vi "Microscopy.Acquisition Engine.vi"(5 "Acquisition Parameters":T4, 6 "Trig Offset":u8, 7 "Reset?":bool, 8 "Data Valid In":bool, 9 "Reference Trigger Edge?":bool, 10 "Arm Acquisition Engine":bool, 11 "Channel Data In":T3=[0, 0, 0, 0]) -> (0 "Data Valid Out":bool, 1 "Read from Buffer":bool, 2 "Acquisition Status":T1={"Reset"=FALSE, "Acquisition Engine Start (Arm)"=FALSE, "Current State"=enum."Acquire Pre-Trigger Samples", "Trig Offset"=0, "Points Unread"=0, "Points Acquired"=0, "Records Done"=0, "Start of Read"=FALSE, "End of Read"=FALSE, "Start of Record"=FALSE, "End of Record"=FALSE, "Ready for Ref Trig"=FALSE, "In Reset?"=FALSE}, 3 "Channel Data Out":T3, 4 "Ready for Ref Trig":bool)   [LabVIEW 2012]
doc: "This VI executes the state machine of the acquisition engine."
uses:
  Acquisition Parameters.ctl
  Multi-Channel Analog Input Data.ctl
  Acquisition Status.ctl
  Acquisition Engine State.ctl
panel:
  in  "Re-Arm Ticks to Wait":u16=3
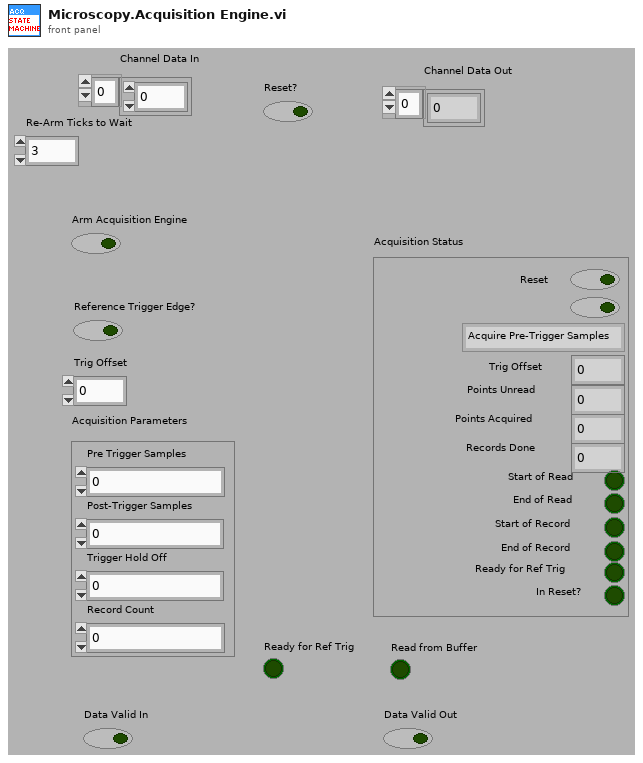
[diagram p1: front panel]
types:
  T1 = typedef "Acquisition Status.ctl" = cluster{"Reset":bool, "Acquisition Engine Start (Arm)":bool, "Current State":T2, "Trig Offset":u8, "Points Unread":u16, "Points Acquired":u16, "Records Done":u16, "Start of Read":bool, "End of Read":bool, "Start of Record":bool, "End of Record":bool, "Ready for Ref Trig":bool, "In Reset?":bool}
  T2 = typedef "Acquisition Engine State.ctl" = enum8{"Idle", "Arm Acquisition Engine", "Acquire Pre-Trigger Samples", "Wait for Trigger", "Acquisition Hold Off Time", "Read Data from Buffer", "Check Records Done?", "Re-Arm State", "Flush Available Data"}
  T3 = typedef "Multi-Channel Analog Input Data.ctl" = i16[]
  T4 = typedef "Acquisition Parameters.ctl" = cluster{"Pre Trigger Samples":u16, "Post-Trigger Samples":u16, "Trigger Hold Off":u16, "Record Count":u16}
  T5 = typedef "State Execution Output.ctl" = cluster{"Ready for Ref Trig?":bool, "End of Record":bool, "Start of Read":bool, "Points in Circular Buffer":u16, "Decrement Points in Circular Buffer":bool, "Read Point from Buffer":bool}
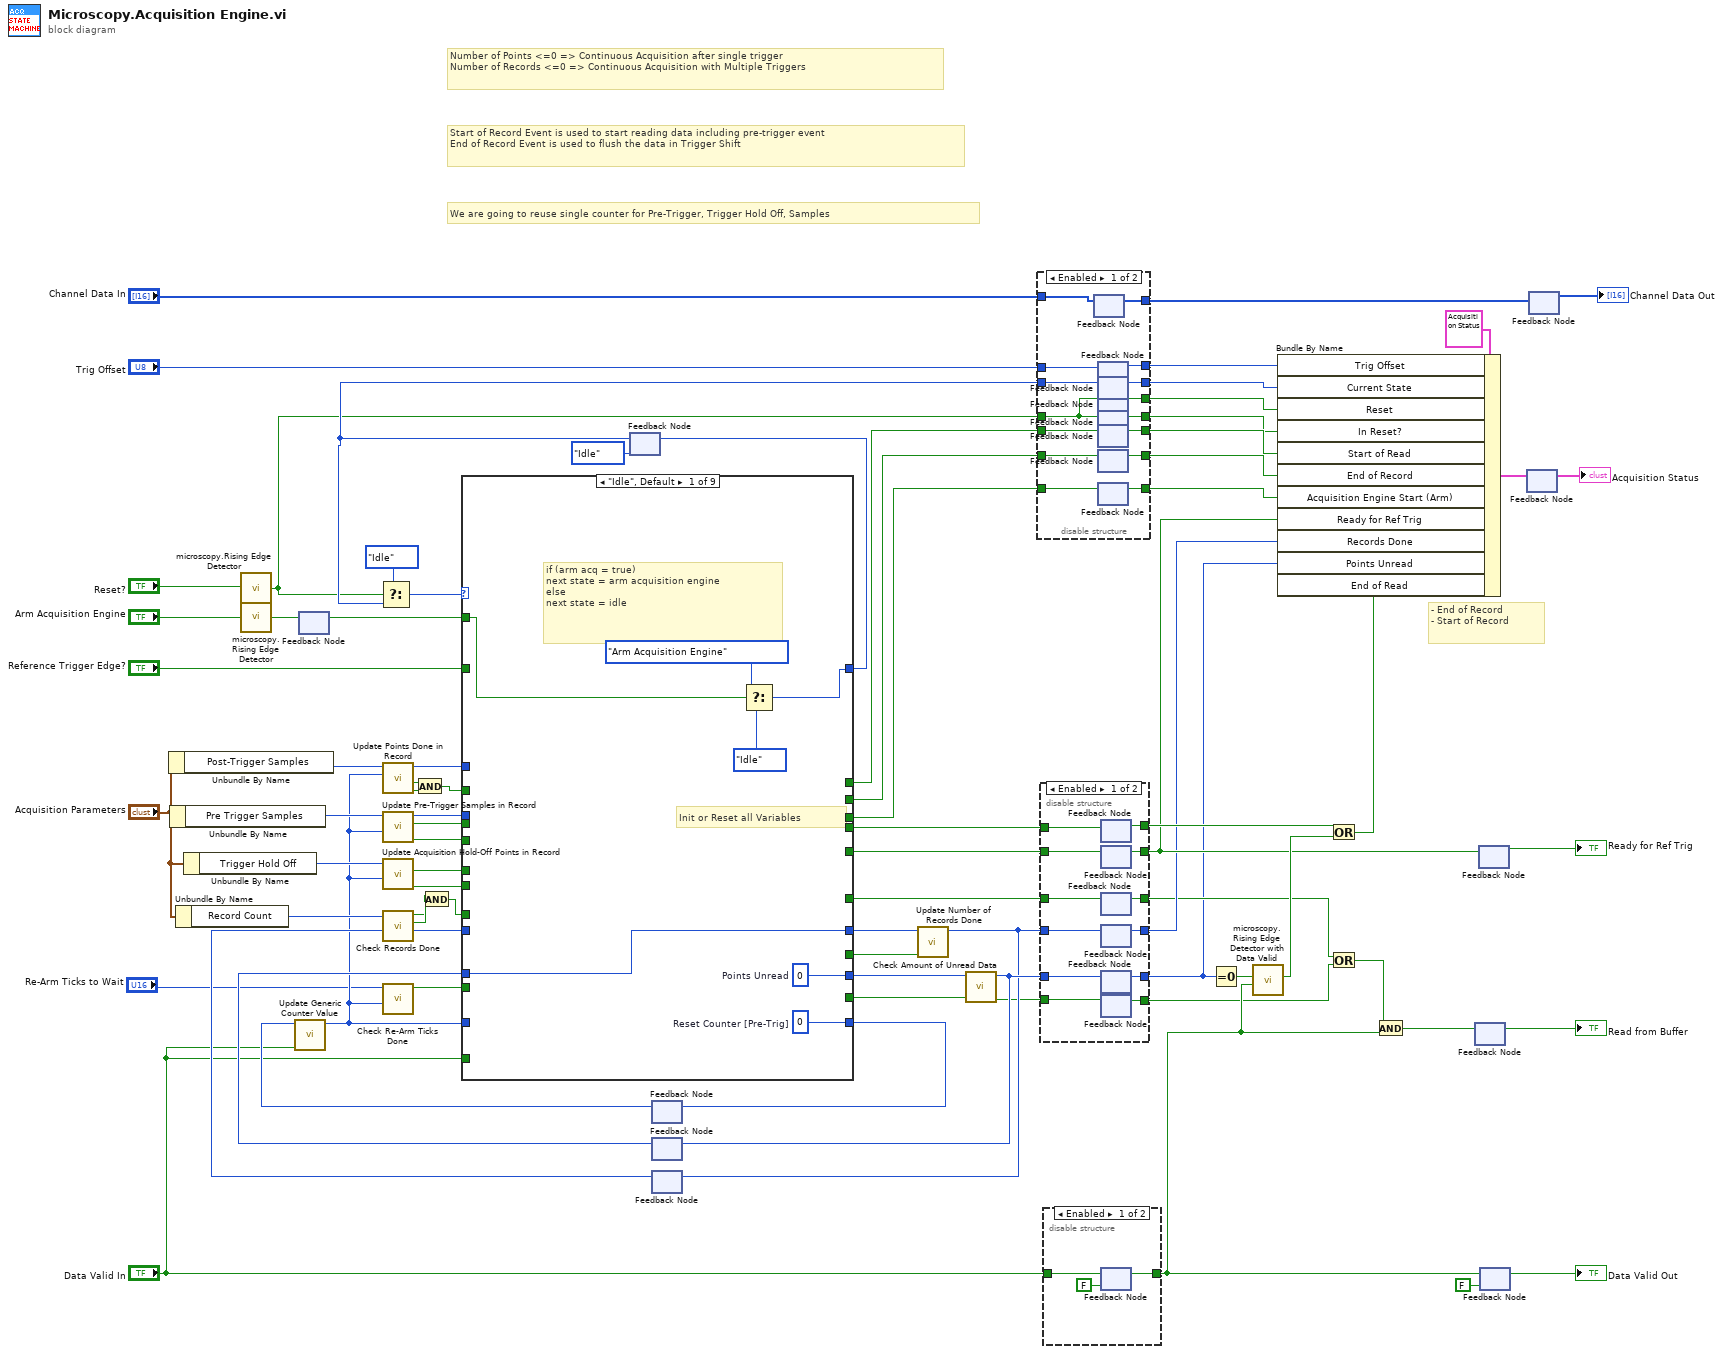
[diagram p0: block diagram]
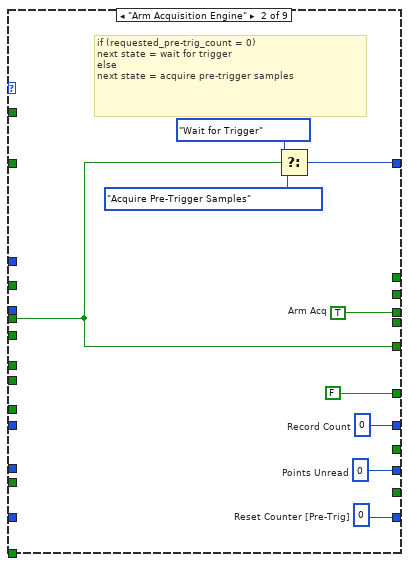
[diagram p5: hidden frame]
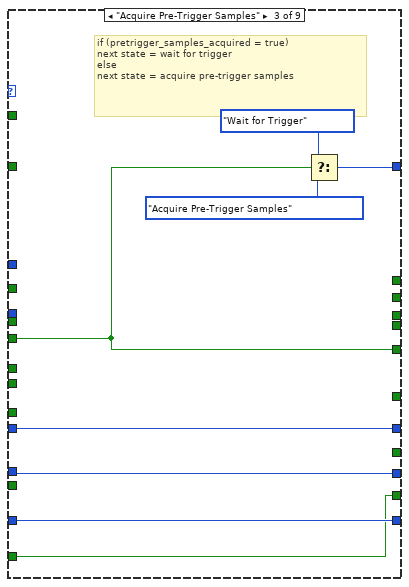
[diagram p6: hidden frame]
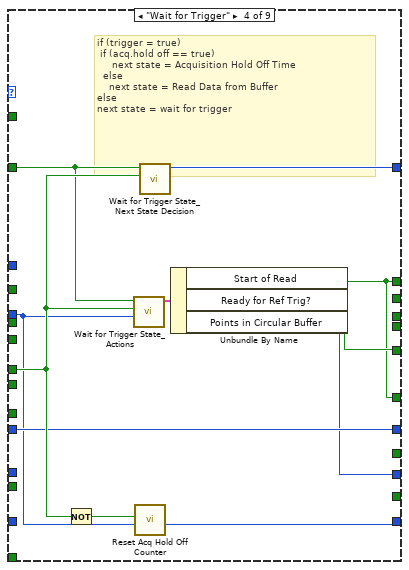
[diagram p7: hidden frame]
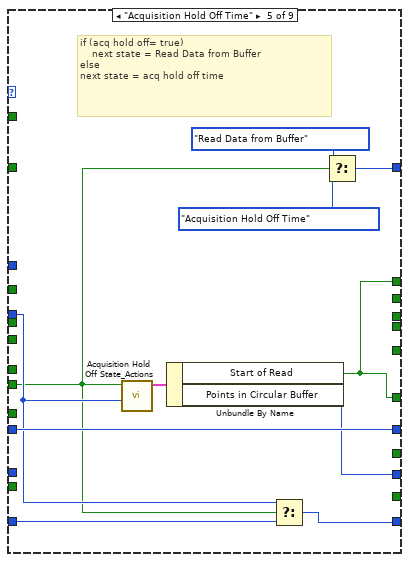
[diagram p8: hidden frame]
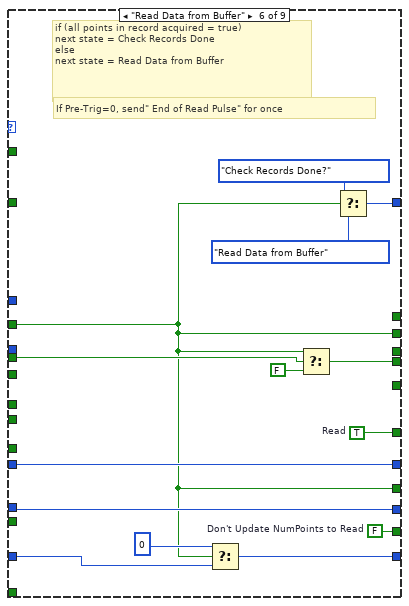
[diagram p9: hidden frame]
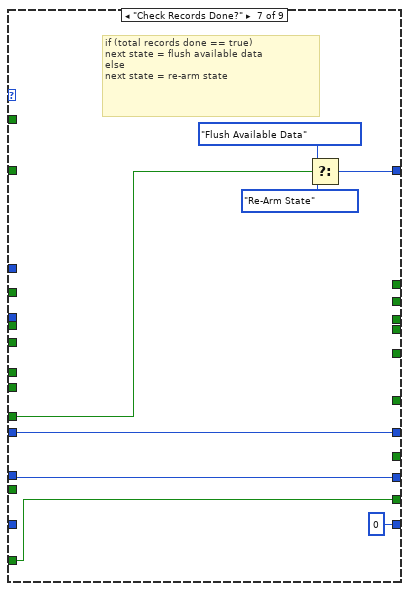
[diagram p10: hidden frame]
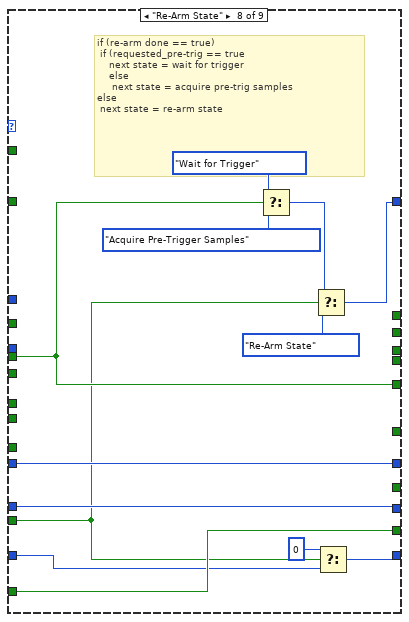
[diagram p11: hidden frame]
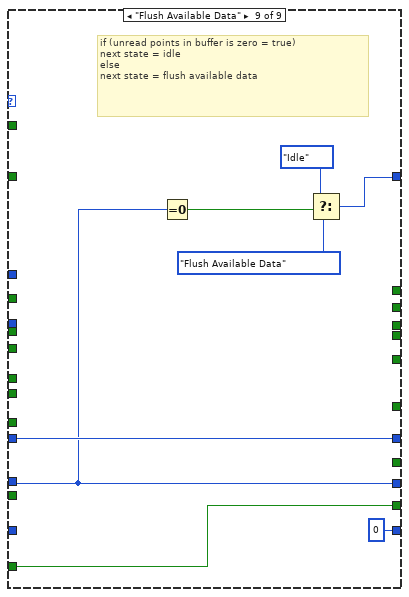
[diagram p12: hidden frame]
diagram:
  # "Number of Points <=0 => Continuous Acquisition after single trigger\nNumber of Records <=0 => Continuous Acquisition with Multiple Triggers"
  # "- End of Record\n- Start of Record"
  # "Start of Record Event is used to start reading data including pre-trigger event\nEnd of Record Event is used to flush the data in Trigger Shift"
  # "We are going to reuse single counter for Pre-Trigger, Trigger Hold Off, Samples"
  n1 = Unbundle By Name("Acquisition Parameters") -> ("Post-Trigger Samples"=w42:u16)
  n2 = Unbundle By Name("Acquisition Parameters") -> ("Pre Trigger Samples"=w61:u16)
  n3 = Unbundle By Name("Acquisition Parameters") -> ("Record Count"=w59:u16)
  n4 = Unbundle By Name("Acquisition Parameters") -> ("Trigger Hold Off"=w69:u16)
  n5 = call "microscopy.Rising Edge Detector.vi"("signal"="Reset?") -> ("edge detected"=w45:bool)  [unwired: 14 in]
  n6 = call "microscopy.Rising Edge Detector.vi"("signal"="Arm Acquisition Engine") -> ("edge detected"=w78:bool)  [unwired: 14 in]
  n7 = feedback-in #1(w78) -> ()
  n8 = feedback #1() -> (w2:bool)  [unwired: 1 in]
  n9 = feedback #2(Acquisition_Engine_State."Idle" ("f")) -> (w51:T2)
  n10 = Select(t=Acquisition_Engine_State."Idle" ("f"), s=w45, f=w51) -> (s? t:f=w75:T2)
  n11 = feedback #3() -> (w74:u16)  [unwired: 1 in]
  n12 = call "Update Generic Counter Value.vi"("Increment?"="Data Valid In", "Input Counter Val"=w74) -> ("Updated Counter Val"=w44:u16)  [unwired: 9 in]
  n13 = call "Update Points Done in Record.vi"("Points Acquired"=w44, "Points to Acquire"=w42) -> ("Points Done ?"=w34:bool, "Points to Acquire > 0?"=w29:bool, "Updated Points Acquired"=w35:u16)  [unwired: 7 in]
  n14 = call "Update Pre-Trigger Samples in Record.vi"("Pre-Trigger Samples Acquired"=w44, "Pre-Trigger Samples to Acquire"=w61) -> ("Pre-Trigger Samples Done ?"=w72:bool, "Is Pre-Trig =0?"=w73:bool, "Pre-Trigger Samples to Acquire"=w50:u16)  [unwired: 6 in, 1 out]
  n15 = call "Update Acquisition Hold-Off Points in Record.vi"("Trigger Hold Off Ticks Finished"=w44, "Trigger Hold-Off Ticks"=w69) -> ("Trigger Hold Off Ticks Finish"=w70:bool, "Is Trigger Hold Off =0?"=w71:bool)  [unwired: 7 in, 1 out]
  n16 = call "Check Re-Arm Ticks Done.vi"("Re-Arm Ticks"=w44, "Re-Arm Ticks to Wait"="Re-Arm Ticks to Wait") -> ("Re-Arm Ticks Done?"=w43:bool)  [unwired: 8 in, 1 out]
  n17 = And(x=w29, y=w34) -> (x .and. y?=w33:bool)
  n18 = feedback #4() -> (w63:u16)  [unwired: 1 in]
  n19 = feedback #5() -> (w66:u16)  [unwired: 1 in]
  n20 = call "Check Records Done.vi"("Records Finished"=w66, "Records to Acquire"=w59) -> ("Updated Records Finished"=w65:u16, "Is NumRecords >0?"=w31:bool, "Records Done?"=w30:bool)  [unwired: 7 in]
  n21 = And(x=w30, y=w31) -> (x .and. y?=w32:bool)
  n22 = case shown="\"Idle\", Default" w75 {
    tunnel: [w87 w88 w102 w114 w126 w139 w146 w153 w168] -> w54
    tunnel: "Reference Trigger Edge?" -> [_ _ _ w107 _ _ _ _ _]
    tunnel: w72 -> [_ _ w98 _ _ _ _ _ _]
    tunnel: w33 -> [_ _ _ _ _ w129 _ _ _]
    tunnel: w2 -> [w82 _ _ _ _ _ _ _ _]
    tunnel: [_ _ _ _ _ w129 _ _ _] -> w53
    tunnel: w73 -> [_ w89 _ _ _ w130 _ w157 _]
    tunnel: w70 -> [_ _ _ _ w117 _ _ _ _]
    tunnel: w71 -> [_ _ _ w113 _ _ _ _ _]
    tunnel: [w81 w94 w101 w112 w123 w137 w145 w159 w169] -> w68
    tunnel: [_ _ _ _ _ w129 _ _ _] -> w67
    tunnel: w65 -> [_ _ w101 w112 w123 w137 w145 w159 w169]
    tunnel: w32 -> [_ _ _ _ _ _ w143 _ _]
    tunnel: w44 -> [_ _ w100 _ w122 w131 _ w151 _]
    tunnel: [w84 w93 w100 w115 w121 w133 u16 0 ("Updated Records Done") w152 u16 0 ("Updated Records Done")] -> w64
    tunnel: w50 -> [_ _ _ w108 w118 _ _ _ _]
    tunnel: [w83 w92 w99 w111 w119 w136 w144 w158 w165] -> w11
    tunnel: w63 -> [w81 _ w99 _ _ w136 w144 w158 w165]
    tunnel: [_ _ w97 _ _ w135 w141 w156 w162] -> w62
    tunnel: [_ w91 _ _ _ _ _ _ _] -> w58
    tunnel: [_ FALSE _ w105 w116 w132 _ _ _] -> w55
    tunnel: [_ w89 w98 w110 _ _ _ w157 _] -> w52
    tunnel: [_ _ _ w105 w116 _ _ _ _] -> w46
    tunnel: "Data Valid In" -> [_ _ w97 _ _ _ w141 w156 w162]
    tunnel: w43 -> [_ _ _ _ _ _ _ w150 _]
    tunnel: [_ _ _ _ _ w127 _ _ _] -> w38
    tunnel: w35 -> [_ _ _ _ _ _ _ _ _]
    frame "Idle", Default {
      w83 = u16 0  # Points Unread
      w84 = u16 0  # Reset Counter [Pre-Trig]
      # "if (arm acq = true)\nnext state = arm acquisition engine\nelse\nnext state = idle"
      # "Init or Reset all Variables"
      n23 = Select(t=Acquisition_Engine_State."Arm Acquisition Engine" ("f"), s=w82, f=Acquisition_Engine_State."Idle") -> (s? t:f=w87:T2)
    }
    frame "Arm Acquisition Engine" {
      w91 = TRUE  # Arm Acq
      w92 = u16 0  # Points Unread
      w93 = u16 0  # Reset Counter [Pre-Trig]
      w94 = u16 0  # Record Count
      # "if (requested_pre-trig_count = 0)\nnext state = wait for trigger\nelse\nnext state = acquire pre-trigger samples"
      n24 = Select(t=Acquisition_Engine_State."Wait for Trigger" ("f"), s=w89, f=Acquisition_Engine_State."Acquire Pre-Trigger Samples") -> (s? t:f=w88:T2)
    }
    frame "Acquire Pre-Trigger Samples" {
      # "if (pretrigger_samples_acquired = true)\nnext state = wait for trigger\nelse\nnext state = acquire pre-trigger samples"
      n25 = Select(t=Acquisition_Engine_State."Wait for Trigger" ("Acquisition Engine State"), s=w98, f=Acquisition_Engine_State."Acquire Pre-Trigger Samples") -> (s? t:f=w102:T2)
    }
    frame "Wait for Trigger" {
      # "if (trigger = true)\n if (acq.hold off == true)\n     next state = Acquisition Hold Off Time\n  else\n    next state = Read Data from Buffer \nelse\nnext state = wait for trigger"
      n26 = Not(x=w113) -> (.not. x?=w106:bool)
      n27 = call "Wait for Trigger State_Actions.vi"("Pre-Trigger Samples"=w108, "Acq Hold=0?"=w113, "Reference Trigger"=w107) -> ("State Execution Outputs"=w109:T5)  [unwired: 8 in]
      n28 = call "Reset Acq Hold Off Counter.vi"("Value"=w108, "Reset"=w106) -> ("Value"=w115:u16)  [unwired: 9 in]
      n29 = call "Wait for Trigger State_Next State Decision.vi"("Acq Hold=0?"=w113, "Reference Trigger"=w107) -> ("Next State"=w114:T2)  [unwired: 9 in]
      n30 = Unbundle By Name(w109) -> ("Start of Read"=w105:bool, "Ready for Ref Trig?"=w110:bool, "Points in Circular Buffer"=w111:u16)
    }
    frame "Acquisition Hold Off Time" {
      # "if (acq hold off= true)\n    next state = Read Data from Buffer\nelse\nnext state = acq hold off time"
      n31 = call "Acquisition Hold Off State_Actions.vi"("Pre-Trigger Samples"=w118, "Hold-Off Time Done?"=w117) -> ("State Output"=w120:T5)  [unwired: 9 in]
      n32 = Unbundle By Name(w120) -> ("Start of Read"=w116:bool, "Points in Circular Buffer"=w119:u16)
      n33 = Select(t=w118, s=w117, f=w122) -> (s? t:f=w121:u16)
      n34 = Select(t=Acquisition_Engine_State."Read Data from Buffer" ("f"), s=w117, f=Acquisition_Engine_State."Acquisition Hold Off Time") -> (s? t:f=w126:T2)
    }
    frame "Read Data from Buffer" {
      w132 = TRUE  # Read
      w135 = FALSE  # Don't Update NumPoints to Read
      # "If Pre-Trig=0, send\" End of Read Pulse\" for once"
      # "if (all points in record acquired = true)\nnext state = Check Records Done\nelse\nnext state = Read Data from Buffer"
      n35 = Select(t=u16 0 ("Updated Records Done"), s=w129, f=w131) -> (s? t:f=w133:u16)
      n36 = Select(t=w129, s=w130, f=FALSE) -> (s? t:f=w127:bool)
      n37 = Select(t=Acquisition_Engine_State."Check Records Done?", s=w129, f=Acquisition_Engine_State."Read Data from Buffer") -> (s? t:f=w139:T2)
    }
    frame "Check Records Done?" {
      # "if (total records done == true)\nnext state = flush available data\nelse\nnext state = re-arm state"
      n38 = Select(t=Acquisition_Engine_State."Flush Available Data" ("f"), s=w143, f=Acquisition_Engine_State."Re-Arm State") -> (s? t:f=w146:T2)
    }
    frame "Re-Arm State" {
      # "if (re-arm done == true)\n if (requested_pre-trig == true\n    next state = wait for trigger\n    else\n     next state = acquire pre-trig samples\nelse\n next state = re-arm state"
      n39 = Select(t=Acquisition_Engine_State."Wait for Trigger" ("f"), s=w157, f=Acquisition_Engine_State."Acquire Pre-Trigger Samples") -> (s? t:f=w155:T2)
      n40 = Select(t=w155, s=w150, f=Acquisition_Engine_State."Re-Arm State") -> (s? t:f=w153:T2)
      n41 = Select(t=u16 0, s=w150, f=w151) -> (s? t:f=w152:u16)
    }
    frame "Flush Available Data" {
      # "if (unread points in buffer is zero = true)\nnext state = idle\nelse\nnext state = flush available data"
      n42 = Equal To 0?(x=w165) -> (x = 0?=w164:bool)
      n43 = Select(t=Acquisition_Engine_State."Idle" ("f"), s=w164, f=Acquisition_Engine_State."Flush Available Data") -> (s? t:f=w168:T2)
    }
  }
  n44 = feedback-in #2(w54) -> ()
  n45 = feedback-in #3(w64) -> ()
  n46 = call "Update Number of Records Done.vi"("Increment?"=w67, "Records Done"=w68) -> ("Updated Records Done"=w28:u16)  [unwired: 9 in]
  n47 = feedback-in #5(w28) -> ()
  n48 = call "Check Amount of Unread Data.vi"("Decrement"=w62, "Current Num Points Unread"=w11) -> ("NumPoinst!=0 before update"=w10:bool, "Updated NumPoints Unread"=w37:u16)  [unwired: 8 in]
  n49 = feedback-in #4(w37) -> ()
  n50 = disable-structure shown="Enabled" {
    disable-tunnel: w58 -> [w184 w185]
    disable-tunnel: w53 -> [w183 w186]
    disable-tunnel: w51 -> [w182 w189]
    disable-tunnel: "Trig Offset" -> [w181 w190]
    disable-tunnel: w46 -> [w180 w187]
    disable-tunnel: w45 -> [w179 w188]
    disable-tunnel: [w178 w185] -> w25
    disable-tunnel: [w177 w186] -> w24
    disable-tunnel: [w176 w187] -> w23
    disable-tunnel: [w175 w188] -> w22
    disable-tunnel: [w174 w189] -> w21
    disable-tunnel: [w173 w188] -> w20
    disable-tunnel: [w172 w190] -> w19
    disable-tunnel: [w171 _] -> w4
    disable-tunnel: "Channel Data In" -> [w170 _]
    frame Enabled {
      n51 = feedback #6() -> (w171:T3)  [unwired: 1 in]
      n52 = feedback-in #6(w170) -> ()
      n53 = feedback #7() -> (w172:u8)  [unwired: 1 in]
      n54 = feedback-in #7(w181) -> ()
      n55 = feedback #8() -> (w174:T2)  [unwired: 1 in]
      n56 = feedback-in #8(w182) -> ()
      n57 = feedback #9() -> (w173:bool)  [unwired: 1 in]
      n58 = feedback-in #9(w179) -> ()
      n59 = feedback #10() -> (w175:bool)  [unwired: 1 in]
      n60 = feedback-in #10(w179) -> ()
      n61 = feedback #11() -> (w176:bool)  [unwired: 1 in]
      n62 = feedback-in #11(w180) -> ()
      n63 = feedback #12() -> (w177:bool)  [unwired: 1 in]
      n64 = feedback-in #12(w183) -> ()
      n65 = feedback #13() -> (w178:bool)  [unwired: 1 in]
      n66 = feedback-in #13(w184) -> ()
    }
    frame Disabled {
    }
  }
  n67 = disable-structure shown="Enabled" {
    disable-tunnel: w55 -> [w202 w206]
    disable-tunnel: w52 -> [w201 w207]
    disable-tunnel: w38 -> [w200 w208]
    disable-tunnel: w37 -> [w199 w204]
    disable-tunnel: w28 -> [w198 w205]
    disable-tunnel: [w197 w208] -> w18
    disable-tunnel: [w196 w207] -> w17
    disable-tunnel: [w195 w205] -> w16
    disable-tunnel: [w194 w206] -> w14
    disable-tunnel: [w193 w204] -> w12
    disable-tunnel: w10 -> [w192 w203]
    disable-tunnel: [w191 w203] -> w9
    frame Enabled {
      n68 = feedback #14() -> (w197:bool)  [unwired: 1 in]
      n69 = feedback-in #14(w200) -> ()
      n70 = feedback #15() -> (w196:bool)  [unwired: 1 in]
      n71 = feedback-in #15(w201) -> ()
      n72 = feedback #16() -> (w194:bool)  [unwired: 1 in]
      n73 = feedback-in #16(w202) -> ()
      n74 = feedback #17() -> (w195:u16)  [unwired: 1 in]
      n75 = feedback-in #17(w198) -> ()
      n76 = feedback #18() -> (w193:u16)  [unwired: 1 in]
      n77 = feedback-in #18(w199) -> ()
      n78 = feedback #19() -> (w191:bool)  [unwired: 1 in]
      n79 = feedback-in #19(w192) -> ()
    }
    frame Disabled {
    }
  }
  n80 = disable-structure shown="Enabled" {
    disable-tunnel: "Data Valid In" -> [w211 w212]
    disable-tunnel: [w210 w212] -> w15
    frame Enabled {
      n81 = feedback #20(FALSE ("Data Valid In")) -> (w210:bool)
      n82 = feedback-in #20(w211) -> ()
    }
    frame Disabled {
    }
  }
  n83 = Equal To 0?(x=w12) -> (x = 0?=w13:bool)
  n84 = call "microscopy.Rising Edge Detector with Data Valid.vi"("Data Valid"=w15, "signal"=w13) -> ("edge detected"=w39:bool)  [unwired: 9 in]
  n85 = Or(x=w18, y=w39) -> (x .or. y?=w36:bool)
  n86 = Bundle By Name(cluster=T1 {"Reset"=FALSE, "Acquisition Engine Start (Arm)"=FALSE, "Current State"=enum."Idle", "Trig Offset"=0, "Points Unread"=0, "Points Acquired"=0, "Records Done"=0, "Start of Read"=FALSE, "End of Read"=FALSE, "Start of Record"=FALSE, "End of Record"=FALSE, "Ready for Ref Trig"=FALSE, "In Reset?"=FALSE} ("Acquisition Status In"), "Trig Offset"=w19, "Current State"=w21, "Reset"=w20, "In Reset?"=w22, "Start of Read"=w23, "End of Record"=w24, "Acquisition Engine Start (Arm)"=w25, "Ready for Ref Trig"=w17, "Records Done"=w16, "Points Unread"=w12, "End of Read"=w36) -> (w57:T1)
  n87 = Or(x=w14, y=w9) -> (x .or. y?=w41:bool)
  n88 = And(x=w41, y=w15) -> (x .and. y?=w47:bool)
  n89 = feedback-in #21(w47) -> ()
  n90 = feedback #21() -> (→"Read from Buffer":bool)  [unwired: 1 in]
  n91 = feedback-in #22(w17) -> ()
  n92 = feedback #22() -> (→"Ready for Ref Trig":bool)  [unwired: 1 in]
  n93 = feedback-in #23(w15) -> ()
  n94 = feedback #23(FALSE ("Data Valid In")) -> (→"Data Valid Out":bool)
  n95 = feedback-in #24(w57) -> ()
  n96 = feedback #24() -> (→"Acquisition Status":T1)  [unwired: 1 in]
  n97 = feedback-in #25(w4) -> ()
  n98 = feedback #25() -> (→"Channel Data Out":T3)  [unwired: 1 in]
